vi "Lock_in_single_meas.vi"(10 "Lock-in-Amplifier VISA":refnum<visa-resource-name>) -> (0 "error out":errorcluster, 1 "Lockin_phas":dbl, 2 "Lockin_ampl":dbl, 3 "Freq":dbl)   [LabVIEW 2015]
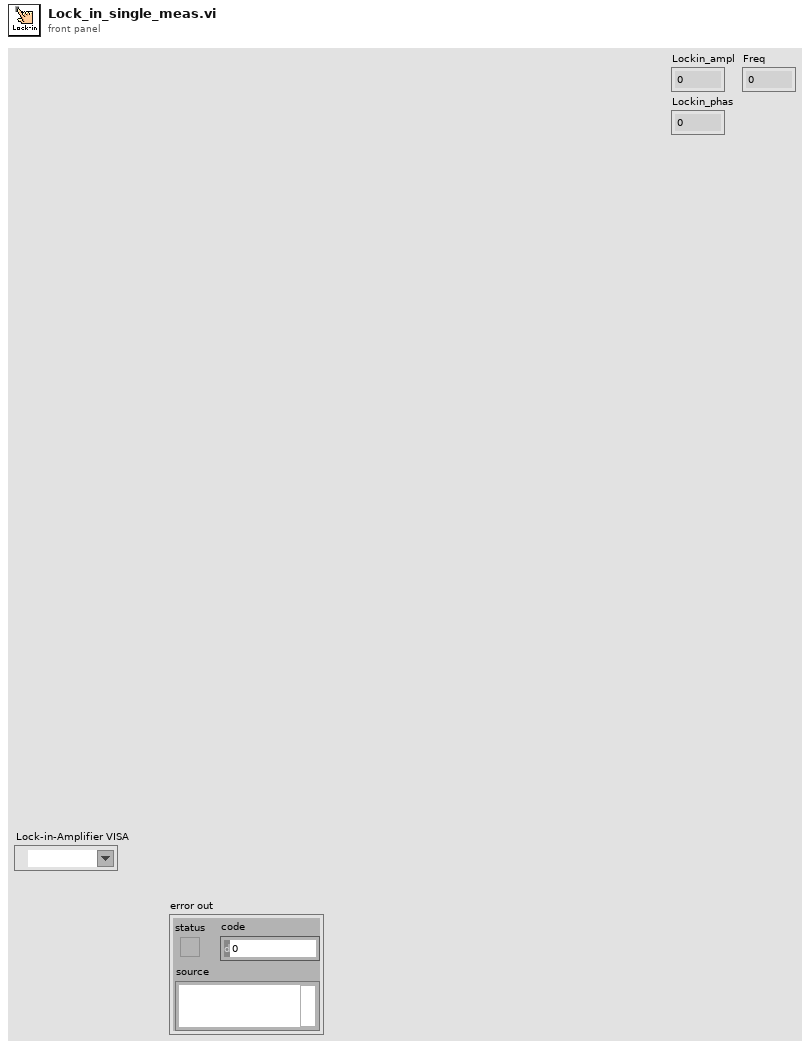
[diagram p1: front panel]
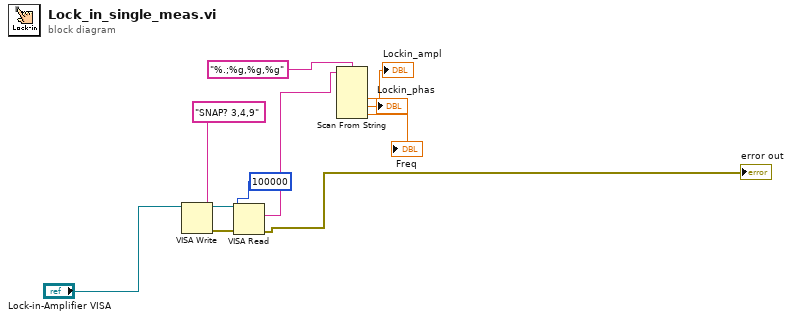
[diagram p0: block diagram]
diagram:
  n1 = VISA Write(VISA resource name="Lock-in-Amplifier VISA", write buffer="SNAP? 3,4,9") -> (VISA resource name out=w6:refnum<visa-resource-name>, error out=w5:errorcluster)  [unwired: 1 in, 1 out]
  n2 = VISA Read(VISA resource name=w6, byte count=u32 100000, error in (no error)=w5) -> (read buffer=w10:string, error out=→"error out":errorcluster)  [unwired: 2 out]
  n3 = Scan From String(format string="%.;%g,%g,%g", input string=w10) -> (output 1=→"Lockin_ampl":dbl, output 2=→"Lockin_phas":dbl, output 3=→"Freq":dbl)  [unwired: 5 in, 3 out]
